vi "set_triggerable.vi"(8 "error in (no error)":errorcluster, 10 "triggerable?":bool, 11 "DAQ_DL091205Readers in":refnum<class "DAQ_DL091205Readers.lvclass">) -> (0 "error out":errorcluster, 3 "DAQ_DL091205Readers out":refnum<class "DAQ_DL091205Readers.lvclass">)   [LabVIEW 2010, in "DAQ_DL091205Readers.lvclass"]
uses:
  DAQ_DL091205Readers.lvclass
  DAQ_DL091205Readers.lvclass/DAQ_DL091205Readers.ctl
  SignalReader/GenericSignalReader/GenericSignalReader/GenericSignalReader.lvclass
  DAQ_DL090211Scaffold/DAQ_DL090211Scaffold/DAQ_DL090211Scaffold.lvclass
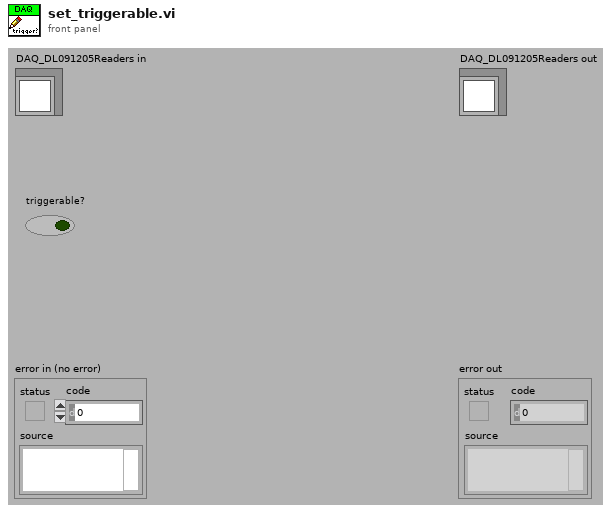
[diagram p1: front panel]
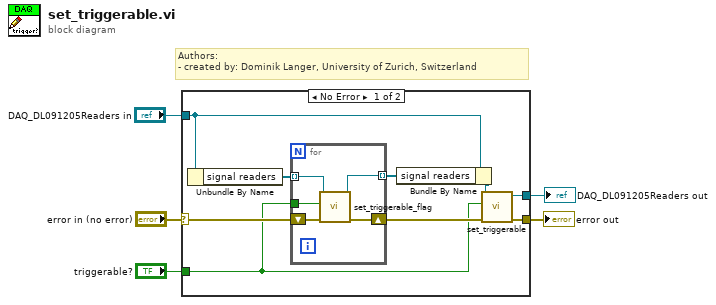
[diagram p0: block diagram]
diagram:
  # "Authors: \n- created by: Dominik Langer, University of Zurich, Switzerland"
  n1 = case shown="No Error" "error in (no error)" {
    selector: "error in (no error)" -> [w9 w20]
    tunnel: [w14 w20] -> w5
    tunnel: [w13 w21] -> w4
    tunnel: "triggerable?" -> [w7 _]
    tunnel: "DAQ_DL091205Readers in" -> [w12 w21]
    frame No Error {
      n2 = Unbundle By Name(w12) -> ("signal readers"=w10:refnum<class "GenericSignalReader.lvclass">[])
      n3 = for {
        tunnel: w10 -> [w16] mode=indexing
        shift-right: [w18] -> w8
        shift-left: w9 -> [w19]
        tunnel: w7 -> [w17]
        tunnel: [w15] -> w6 mode=indexing
        n4 = call-dynamic "set_triggerable_flag.vi"("error in (no error)"=w19, "triggerable?"=w17, "GenericSignalReader in"=w16) -> ("error out"=w18:errorcluster, "GenericSignalReader out"=w15:refnum<class "GenericSignalReader.lvclass">)  [unwired: 7 in]
      }
      n5 = Bundle By Name(cluster=w12, "signal readers"=w6) -> (w11:refnum<class "DAQ_DL091205Readers.lvclass">)
      n6 = call-parent "set_triggerable.vi"("error in (no error)"=w8, "triggerable?"=w7, "GenericDAQ in"=w11) -> ("error out"=w14:errorcluster, "GenericDAQ out"=w13:refnum<class "DAQ_DL091205Readers.lvclass">)  [unwired: 7 in]
    }
    frame Error {
    }
  }
  "error out" <- w5
  "DAQ_DL091205Readers out" <- w4
